vi "Create StaticVIRefnum Job.vi"(5 "Job.StaticVIRef in":refnum<class "Job.StaticVIRef.lvclass">, 7 "Job Name":string, 8 "error in (no error)":errorcluster, 9 "Output Terminal Name (stdout)":string="stdout", 10 "Input Terminal Name (stdin)":string="stdin", 11 "Static VI Refnum":refnum<vi>) -> (0 "error out":errorcluster, 3 "Job.StaticVIRef out":refnum<class "Job.StaticVIRef.lvclass">)   [LabVIEW 2013, in "openCronJob.lvlib" / "Job.StaticVIRef.lvclass"]
uses:
  Job.StaticVIRef.lvclass
  Job.StaticVIRef.lvclass/Job.StaticVIRef.ctl
  Job/Job.lvclass
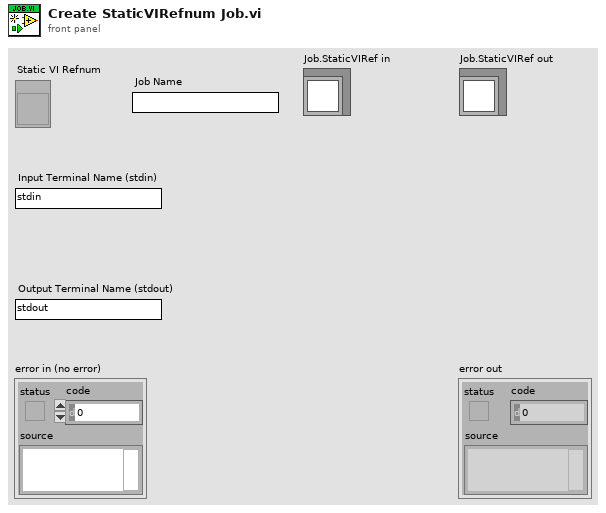
[diagram p1: front panel]
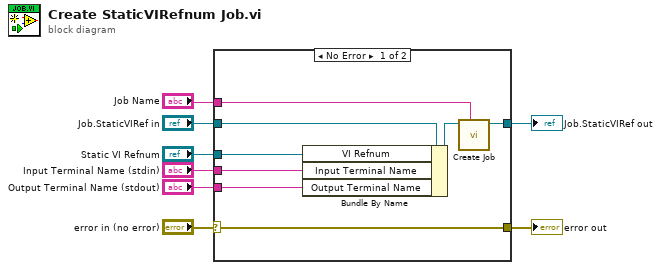
[diagram p0: block diagram]
diagram:
  n1 = case shown="No Error" "error in (no error)" {
    selector: "error in (no error)" -> [w16 w18]
    tunnel: [w16 w18] -> w7
    tunnel: [w10 w17] -> w5
    tunnel: "Job.StaticVIRef in" -> [w14 w17]
    tunnel: "Static VI Refnum" -> [w15 _]
    tunnel: "Input Terminal Name (stdin)" -> [w13 _]
    tunnel: "Output Terminal Name (stdout)" -> [w12 _]
    tunnel: "Job Name" -> [w9 _]
    frame No Error {
      n2 = Bundle By Name(cluster=w14, "VI Refnum"=w15, "Input Terminal Name"=w13, "Output Terminal Name"=w12) -> (w11:refnum<class "Job.StaticVIRef.lvclass">)
      n3 = call "Create Job.vi"("Job Name"=w9, "Job in"=w11) -> ("Job"=w10:refnum<class "Job.StaticVIRef.lvclass">)  [unwired: 8 in, 1 out]
    }
    frame Error {
    }
  }
  "error out" <- w7
  "Job.StaticVIRef out" <- w5
